vi "Decimate and Interpolate (single).vi"(8 "error in (no error)":errorcluster, 10 "Configure":T1={"X Low"=0.05, "X High"=0.5, "X Step"=0.01, "fake point value"=0.05} {"fake point value" format="%#_6p"; "X Step" format="%#_6p"; "X High" format="%#_6p"; "X Low" format="%#_6p"}, 11 "XY-data in":cluster{"X-array":dbl[], "Y-array":dbl[]}) -> (0 "error out":errorcluster, 3 "XY-data out":cluster{"X-array":dbl[], "Y-array":dbl[]} {"Y-array" format="%.2p"; "X-array" format="%.2p"})   [LabVIEW 2016, in "xy_utilities.lvlib"]
uses:
  xy_utilities.lvlib
  <vilib>/Analysis/baseanly.llb/Mean (DBL).vi
  <vilib>/gmath/NI_Gmath.lvlib
  <vilib>/Analysis/NI_AALBase.lvlib
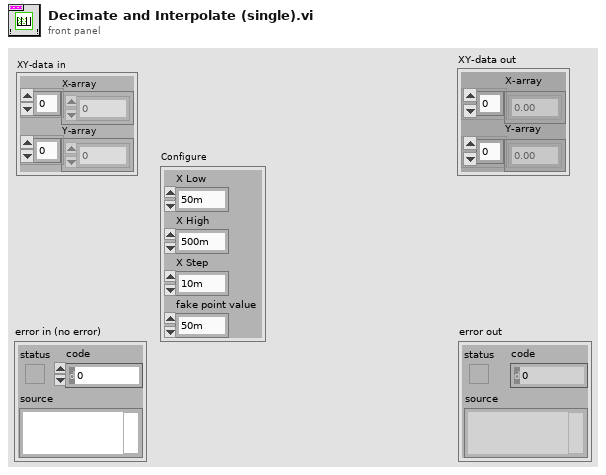
[diagram p1: front panel]
types:
  T1 = cluster{"X Low":dbl, "X High":dbl, "X Step":dbl, "fake point value":dbl}
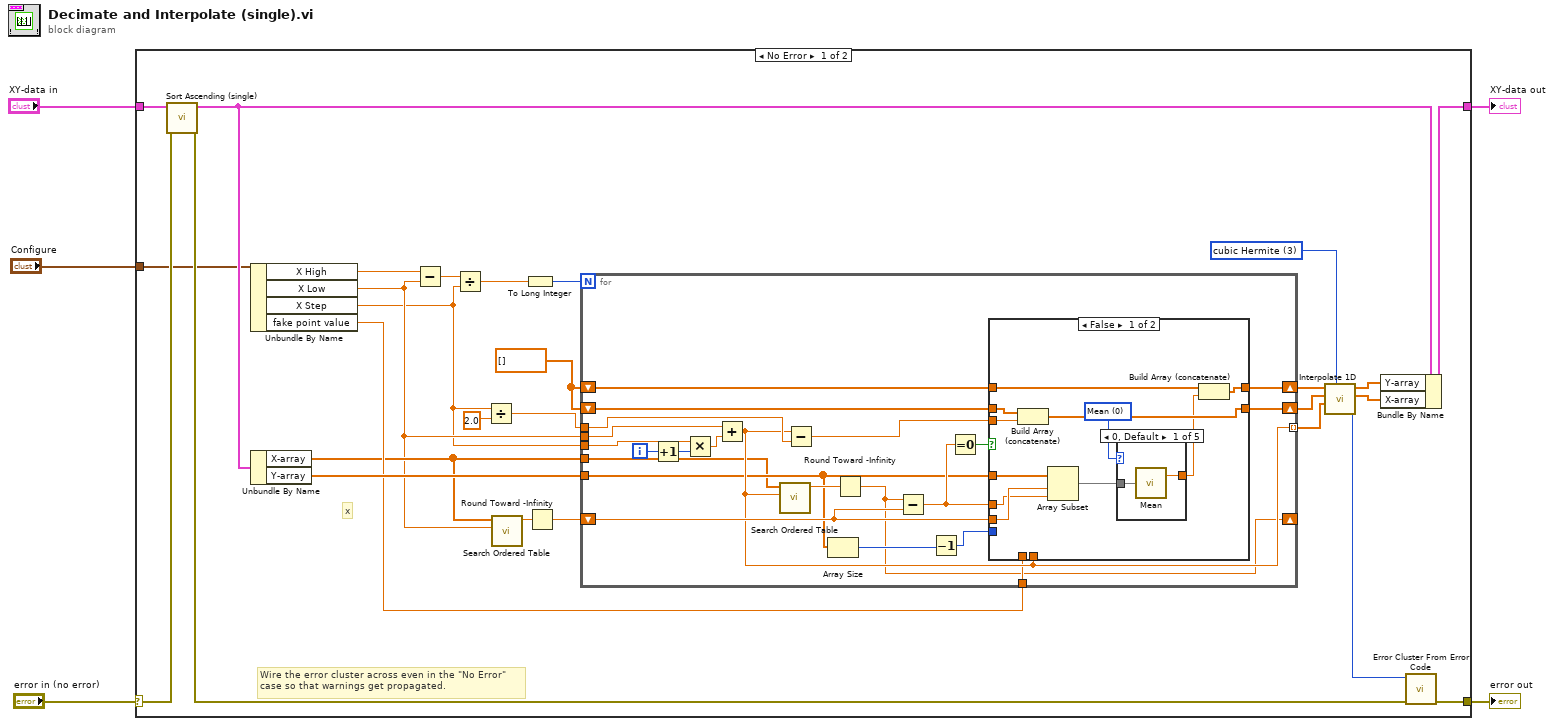
[diagram p0: block diagram]
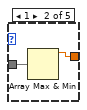
[diagram p2: hidden frame]
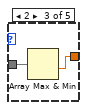
[diagram p3: hidden frame]
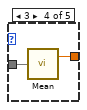
[diagram p4: hidden frame]
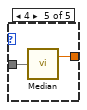
[diagram p5: hidden frame]
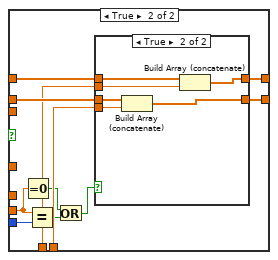
[diagram p6: hidden frame]
diagram:
  n1 = case shown="No Error" "error in (no error)" {
    selector: "error in (no error)" -> [w19 w97]
    tunnel: [w15 w97] -> w4
    tunnel: "XY-data in" -> [w33 w96]
    tunnel: [w21 w96] -> w2
    tunnel: "Configure" -> [w7 _]
    frame No Error {
      w14 = 3 items=["nearest", "linear", "spline", "cubic Hermite", "Lagrange"] ("method")
      w24 = dbl[] []
      # "x"
      # "Wire the error cluster across even in the \"No Error\"\ncase so that warnings get propagated."
      n2 = call "Sort Ascending (single).vi"("error in (no error)"=w19, "XY-data"=w33) -> ("error out"=w16:errorcluster, "Sorted XY-data out"=w11:cluster{"X-array":dbl[], "Y-array":dbl[]})  [unwired: 8 in]
      n3 = Unbundle By Name(w7) -> ("X High"=w20:dbl, "X Low"=w13:dbl, "X Step"=w6:dbl, "fake point value"=w22:dbl)
      n4 = Unbundle By Name(w11) -> ("X-array"=w18:dbl[], "Y-array"=w23:dbl[])
      n5 = Subtract(x=w20, y=w13) -> (x-y=w32:dbl)
      n6 = Divide(x=w32, y=w6) -> (x/y=w29:dbl)
      n7 = Divide(x=w6, y=2.0) -> (x/y=w30:dbl)
      n8 = call <vilib>:"Search Ordered Table.vi"("x value"=w13, "ordered x array"=w18) -> ("fractional index"=w26:dbl)  [unwired: 9 in]
      n9 = To Long Integer(number=w29) -> (32bit integer=w12:i32)
      n10 = Round Toward -Infinity(1:w26) -> (0:w25:dbl)
      n11 = for {
        N: w12 -> [_]
        tunnel: w13 -> [w37]
        tunnel: w6 -> [w34]
        tunnel: w18 -> [w39]
        tunnel: w23 -> [w43]
        shift-right: [w38] -> _
        shift-left: w25 -> [w47]
        tunnel: w30 -> [w53]
        shift-right: [w48] -> w8
        shift-left: w24 -> [w36]
        shift-right: [w45] -> w28
        shift-left: w24 -> [w35]
        tunnel: [w44] -> w27 mode=indexing
        tunnel: w22 -> [w40]
        i -> [w52]
        n12 = Increment(x=w52) -> (x+1=w51:i32)
        n13 = Multiply(x=w34, y=w51) -> (x*y=w54:dbl)
        n14 = Add(x=w37, y=w54) -> (x+y=w44:dbl)
        n15 = call <vilib>:"Search Ordered Table.vi"("x value"=w44, "ordered x array"=w39) -> ("fractional index"=w55:dbl)  [unwired: 9 in]
        n16 = Subtract(x=w44, y=w53) -> (x-y=w49:dbl)
        n17 = Array Size(array=w43) -> (size(s)=w42:i32)
        n18 = Round Toward -Infinity(1:w55) -> (0:w38:dbl)
        n19 = Subtract(x=w38, y=w47) -> (x-y=w46:dbl)
        n20 = Decrement(x=w42) -> (x-1=w41:i32)
        n21 = Equal To 0?(x=w46) -> (x = 0?=w50:bool)
        n22 = case shown="False" w50 {
          tunnel: w49 -> [w66 _]
          tunnel: [w65 w85] -> w48
          tunnel: w36 -> [w64 w87]
          tunnel: w47 -> [w63 w82]
          tunnel: w43 -> [w62 _]
          tunnel: w46 -> [w61 _]
          tunnel: [w58 w83] -> w45
          tunnel: w35 -> [w57 w84]
          tunnel: w44 -> [_ w86]
          tunnel: w41 -> [_ w81]
          tunnel: w40 -> [_ w78]
          frame False {
            w56 = u16 0 items=["Mean", "Max", "Min", "Sigma", "Median"] ("Method")
            n23 = Build Array (concatenate)(w64, w66) -> (w65:dbl[])
            n24 = Array Subset(array=w62, index=w63, length=w61) -> (w60:dbl[])
            n25 = case shown="0, Default" w56 {
              tunnel: [w68 w70 w72 w74 w75] -> w59
              tunnel: w60 -> [w67 w69 w71 w73 w76]
              frame 0, Default {
                n26 = call-poly <vilib>:"Mean.vi"("X"=w67) -> ("mean"=w68:dbl)  [unwired: 1 out]
              }
              frame 1 {
                n27 = Array Max & Min(array=w69) -> (max value=w70:dbl)  [unwired: 3 out]
              }
              frame 2 {
                n28 = Array Max & Min(array=w71) -> (min value=w72:dbl)  [unwired: 3 out]
              }
              frame 3 {
                n29 = call-poly <vilib>:"Mean.vi"("X"=w73) -> ("mean"=w74:dbl)  [unwired: 1 out]
              }
              frame 4 {
                n30 = call <vilib>:"Median.vi"("X"=w76) -> ("median"=w75:dbl)  [unwired: 1 out]
              }
            }
            n31 = Build Array (concatenate)(w57, w59) -> (w58:dbl[])
          }
          frame True {
            n32 = Equal To 0?(x=w82) -> (x = 0?=w80:bool)
            n33 = Equal?(x=w82, y=w81) -> (x = y?=w79:bool)
            n34 = Or(x=w80, y=w79) -> (x .or. y?=w77:bool)
            n35 = case shown="True" w77 {
              tunnel: w87 -> [w89 w90]
              tunnel: w86 -> [_ w95]
              tunnel: [w89 w94] -> w85
              tunnel: w84 -> [w88 w93]
              tunnel: [w88 w92] -> w83
              tunnel: w78 -> [_ w91]
              frame False {
              }
              frame True {
                n36 = Build Array (concatenate)(w90, w95) -> (w94:dbl[])
                n37 = Build Array (concatenate)(w93, w91) -> (w92:dbl[])
              }
            }
          }
        }
      }
      n38 = call <vilib>:"Interpolate 1D.vi"("method"=w14, "xi"=w27, "X"=w8, "Y"=w28) -> ("error"=w17:i32, "xi used"=w9:dbl[], "yi"=w10:dbl[])  [unwired: 5 in]
      n39 = Bundle By Name(cluster=w11, "Y-array"=w10, "X-array"=w9) -> (w21:cluster{"X-array":dbl[], "Y-array":dbl[]})
      n40 = call <vilib>:"Error Cluster From Error Code.vi"("error in (no error)"=w16, "error code (0)"=w17) -> ("error out"=w15:errorcluster)  [unwired: 7 in]
    }
    frame Error {
    }
  }
  "error out" <- w4
  "XY-data out" <- w2
